vi "DefaultFromIni.vi"(8 "error in (no error)":errorcluster, 11 "FitterBase in":refnum<class "FitterBase.lvclass">) -> (0 "error out":errorcluster, 3 "FitterBase out":refnum<class "FitterBase.lvclass">)   [LabVIEW 2018, in "AnalysisPlugins.lvlib" / "FitterBase.lvclass"]
uses:
  FitterBase.lvclass
  C:/Program Files/National Instruments/LabVIEW 2018/user.lib/NIST/BaseClasses/BasePlugin_class/BasePlugin.lvclass
  Y:/Projects/PMUCal/Modules/Analysis/AnalysisPlugins/AnalysisPluginBaseClass/AnalysisPluginsBase.lvclass
  Typedefs/clAnalysisConfig.ctl
  <userlib>/NIST/BaseClasses/BasePlugin_class/BasePlugin.lvclass/BasePlugin.ctl
  AnalysisPluginBaseClass/AnalysisPluginsBase.lvclass/AnalysisPluginsBase.ctl
  <userlib>/NIST/BaseClasses/BasePlugin_class/Accessors/Read PluginIniFilePath.vi
  AnalysisPluginBaseClass/Accessors/Write AnalysisConfig.vi
  AnalysisPluginBaseClass/AnalysisPluginsBase.lvclass
  <vilib>/Utility/config.llb/NI_LVConfig.lvlib
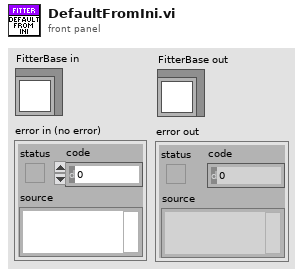
[diagram p1: front panel]
types:
  T1 = typedef "AnalysisPlugins.lvlib/FitterBase.lvclass/clAnalysisConfig.ctl" = cluster{"F0":u32, "SettlingTime":dbl, "AnalysisCycles":dbl, "SampleRate":dbl, "NumChannels":u32, "TsOffset":enum16{"start", "middle", "end"}}
  T2 = typedef "NI_LVConfig.lvlib/Config Data RefNum.ctl" = refnum<k1>
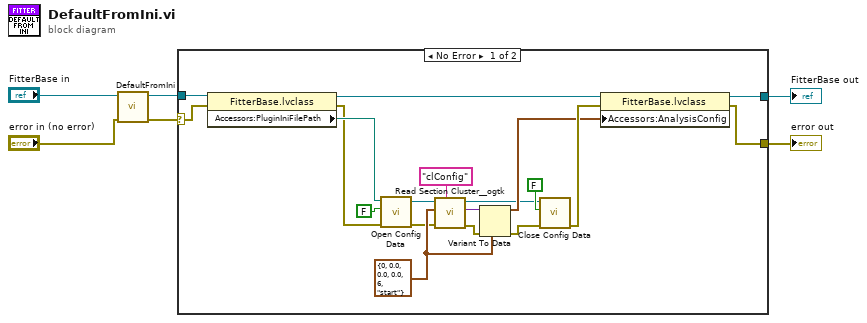
[diagram p0: block diagram]
diagram:
  n1 = call-parent "DefaultFromIni.vi"("error in (no error)"="error in (no error)", "AnalysisPluginsBase in"="FitterBase in") -> ("error out"=w2:errorcluster, "AnalysisPluginsBase out"=w1:refnum<class "FitterBase.lvclass">)  [unwired: 8 in]
  n2 = case shown="No Error" w2 {
    selector: w2 -> [w18 w26]
    tunnel: w1 -> [w19 w27]
    tunnel: [w16 w27] -> w6
    tunnel: [w14 w26] -> w5
    frame No Error {
      w22 = T1 {"F0"=0, "SettlingTime"=0.0, "AnalysisCycles"=0.0, "SampleRate"=0.0, "NumChannels"=6, "TsOffset"=enum."start"} ("clConfig")
      n3 = property class="FitterBase.lvclass"(reference=w19, error in=w18) -> (reference out=w15:refnum<class "FitterBase.lvclass">, error out=w13:errorcluster, "Accessors:PluginIniFilePath"=w17:path)
      n4 = call <vilib>:"Open Config Data.vi"("error in (no error)"=w13, "create file if necessary (T)"=FALSE, "configuration file path"=w17) -> ("error out"=w9:errorcluster, "refnum"=w10:T2)  [unwired: 6 in, 1 out]
      n5 = call <userlib>:"Read Section Cluster__ogtk.vi"("section (optional)"="clConfig", "error in (no error)"=w9, "Section Formatted Cluster Type"=w22, "refnum"=w10) -> ("error out"=w24:errorcluster, "Section Formatted Cluster"=w23:variant, "dup refnum"=w8:T2)  [unwired: 3 in, 2 out]
      n6 = Variant To Data(error in=w24, type=w22, Variant=w23) -> (data=w11:T1, error out=w7:errorcluster)
      n7 = call <vilib>:"Close Config Data.vi"("error in (no error)"=w7, "write file if changed (T)"=FALSE, "refnum"=w8) -> ("error out"=w12:errorcluster)  [unwired: 7 in, 1 out]
      n8 = property class="FitterBase.lvclass"(reference=w15, error in=w12, "Accessors:AnalysisConfig"=w11) -> (reference out=w16:refnum<class "FitterBase.lvclass">, error out=w14:errorcluster)
    }
    frame Error {
    }
  }
  "error out" <- w5
  "FitterBase out" <- w6
